vi "_096.vi"() -> ()   [LabVIEW 2020]
panel:
  out "x/y":dbl
  out "product":i32
  out "sum":i32
  out "result":i32
  in  "Array":dbl[](array[numeric])
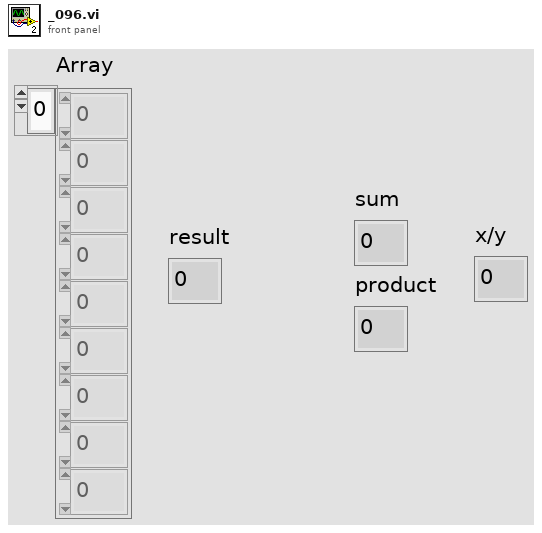
[diagram p1: front panel]
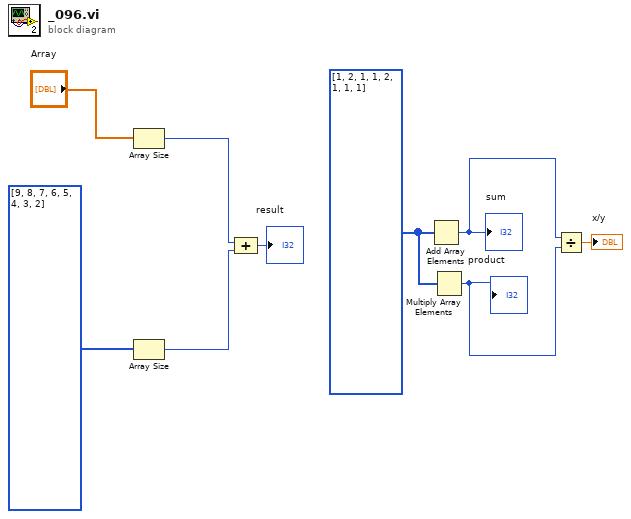
[diagram p0: block diagram]
diagram:
  w4 = i32[] [1, 2, 1, 1, 2, 1, 1, 1]
  n1 = Array Size(array="Array") -> (size(s)=w7:i32)
  n2 = Array Size(array=i32[] [9, 8, 7, 6, 5, 4, 3, 2]) -> (size(s)=w6:i32)
  n3 = Compound Arithmetic op=ADD(w7, w6) -> (→"result":i32)
  n4 = Add Array Elements(numeric array=w4) -> (sum=w3:i32)
  "sum" <- w3
  n5 = Multiply Array Elements(1:w4) -> (0:w2:i32)
  "product" <- w2
  n6 = Divide(x=w3, y=w2) -> (x/y=→"x/y":dbl)
